vi "To JSON.vi"(5 "enable LabVIEW extensions? (T)":bool=TRUE, 6 "Pretty Print?":bool, 7 "LVClass Serializer":refnum<class "JSONtext LVClass Serializer.lvclass">, 8 "error in (no error)":errorcluster, 11 "Serializable Account in":refnum<class "Serializable Account.lvclass">) -> (0 "error out":errorcluster, 2 "<JSON>":string, 3 "Serializable Account out":refnum<class "Serializable Account.lvclass">)   [LabVIEW 2017, in "Serializable Account.lvclass"]
doc: "Creates a JSON string from an object."
uses:
  Serializable Account.lvclass
  <vilib>/JDP Science/JSONtext/LVClass Serializer/JSONtext LVClass Serializer.lvclass
  Serializable Account.lvclass/Serializable Account.ctl
  <vilib>/JDP Science/JSONtext/JSONtext.lvlib
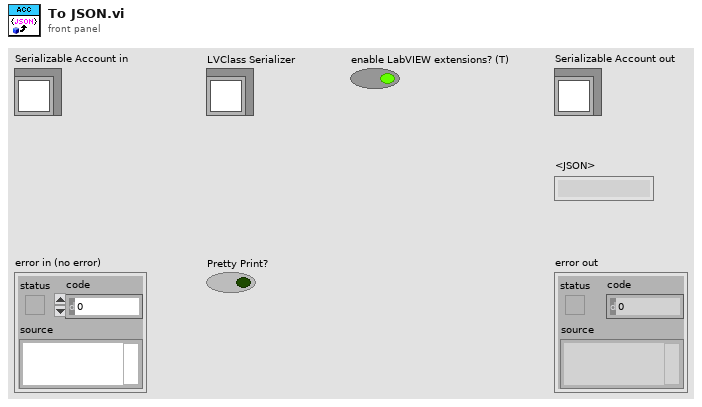
[diagram p1: front panel]
types:
  T1 = cluster{"MD5 message-digest":string, "Email":string, "Active":bool, "CreatedDate":timestamp, "Roles":string[]}
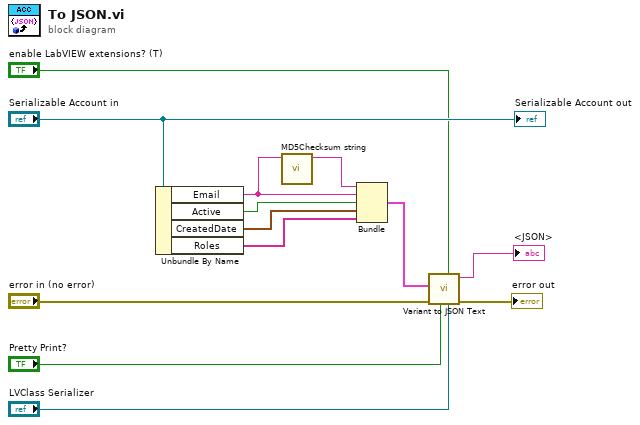
[diagram p0: block diagram]
diagram:
  n1 = Unbundle By Name("Serializable Account in") -> ("Email"=w2:string, "Active"=w10:bool, "CreatedDate"=w11:timestamp, "Roles"=w12:string[])
  n2 = call <vilib>:"MD5Checksum string.vi"("Message String"=w2) -> ("MD5 message-digest"=w1:string)  [unwired: 10 in]
  n3 = Bundle("MD5 message-digest"=w1, "Email"=w2, "Active"=w10, "CreatedDate"=w11, "Roles"=w12) -> (w3:T1)  [unwired: 1 in]
  n4 = call <vilib>:"Variant to JSON Text.vi"("LVClass Serializer"="LVClass Serializer", "enable LabVIEW extensions? (T)"="enable LabVIEW extensions? (T)", "Pretty Print?"="Pretty Print?", "error in (no error)"="error in (no error)", "Variant"=w3) -> ("error out"=→"error out":errorcluster, "<JSON>"=→"<JSON>":string)  [unwired: 4 in, 1 out]
  "Serializable Account out" <- "Serializable Account in"
